vi "Initialise Command Writer.vi"(8 "error in (no error)":errorcluster, 11 "IP Address":string) -> (0 "error out":errorcluster, 3 "Refnum out":refnum<k21>)   [LabVIEW 2017]
doc: "Initialises the command writer stream."
uses:
  HostRTCommunication/Command and Parameters.ctl
  HostRTCommunication/Commands.ctl
  <vilib>/dex/Stream Element Allocation Mode.ctl
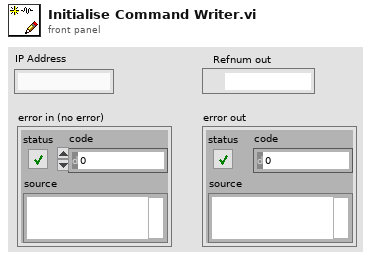
[diagram p1: front panel]
types:
  T1 = typedef "Command and Parameters.ctl" = cluster{"Command":T2, "Command Parameters":variant[]}
  T2 = typedef "Commands.ctl" = enum16{"Set Center Frequency", "Set AGC State", "Set Number Of Averages", "Set Tuner Gain Mode", "Set Frequency Correction", "Set Sample Rate", "Set Manual Gain Value"}
  T3 = typedef "Stream Element Allocation Mode.ctl" = u32
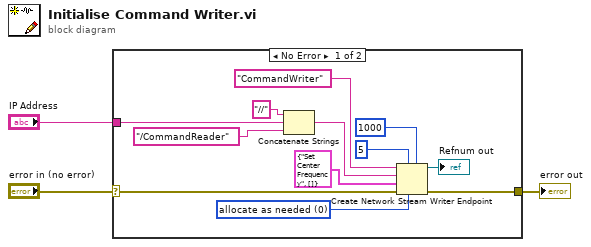
[diagram p0: block diagram]
diagram:
  n1 = case shown="No Error" "error in (no error)" {
    selector: "error in (no error)" -> [w8 w16]
    tunnel: [w14 w16] -> w3
    tunnel: "IP Address" -> [w4 _]
    frame No Error {
      w13 = T3 0 items=["allocate as needed", "pre-allocate"] ("element allocation mode")
      n2 = Concatenate Strings("//" ("string"), w4, "/CommandReader" ("reader url")) -> (w5:string)
      n3 = Create Network Stream Writer Endpoint(5:1000 ("timeout in ms (-1)"), 6:w13, 7:5 ("writer buffer size"), 8:w8, 9:T1 {"Command"=enum."Set Center Frequency", "Command Parameters"=[]} ("Cluster"), 10:w5, 11:"CommandWriter" ("writer name")) -> (0:w14:errorcluster, 3:→"Refnum out":refnum<k21>)
    }
    frame Error {
    }
  }
  "error out" <- w3
